vi "Error Query.vi"(8 "error in (no error)":errorcluster, 11 "VISA resource name":refnum<visa-resource-name>) -> (0 "error out":errorcluster, 1 "Error Message":string, 2 "Error Code":i32[](array[numeric]), 3 "VISA resource name out":refnum<visa-resource-name>)   [LabVIEW 2018, in "Tektronix TDS 200 1000 2000 Series.lvlib"]
doc: "Queries an instrument for any errors in the error queue of the instrument. The Error Query VI continuously reads errors until this VI reads all the errors from the instrument. \n<B>Note</B>: Because most driver VIs automatically call the Error Query VI, you do not need to call this VI in an application."
uses:
  Tektronix TDS 200 1000 2000 Series.lvlib
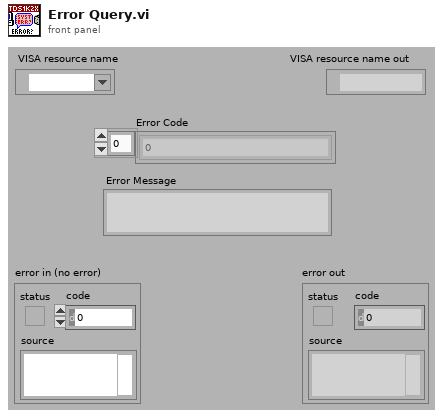
[diagram p1: front panel]
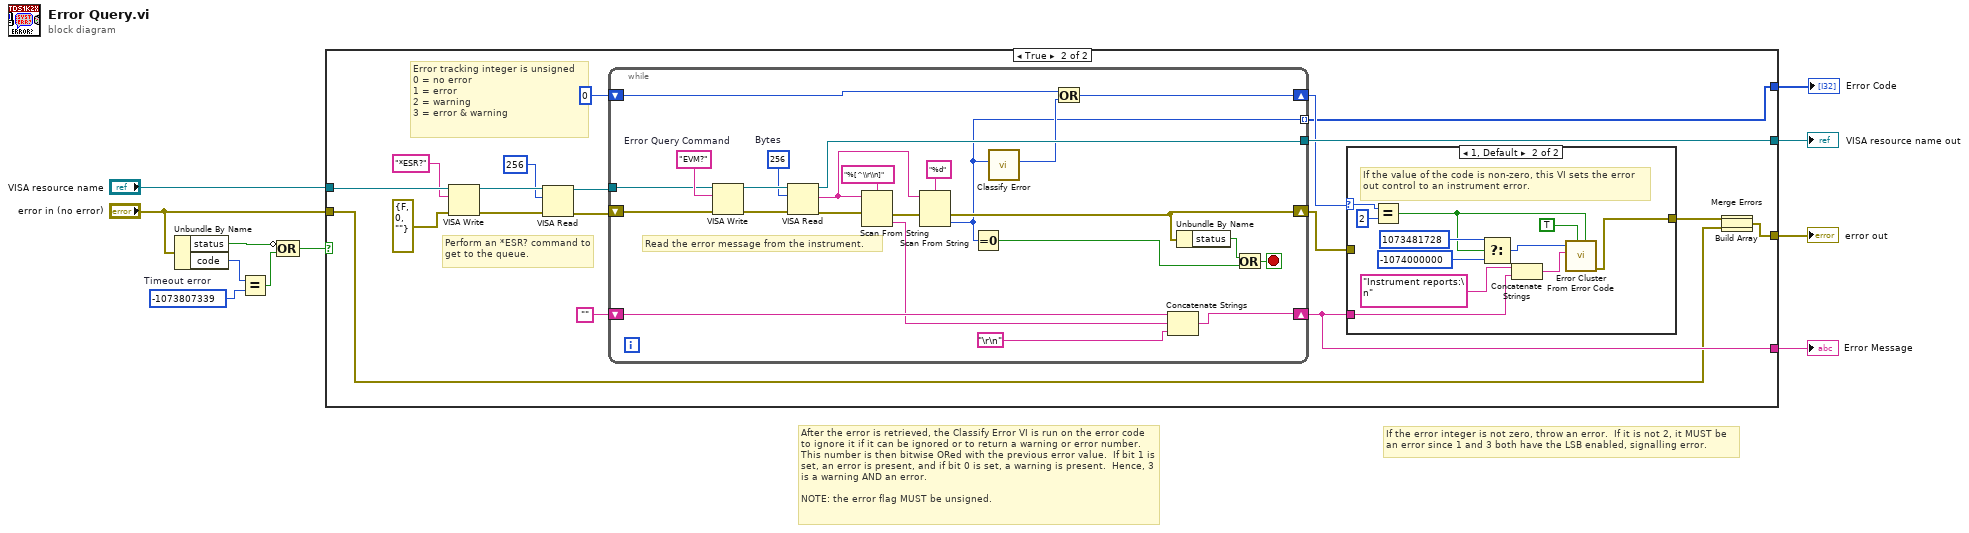
[diagram p0: block diagram]
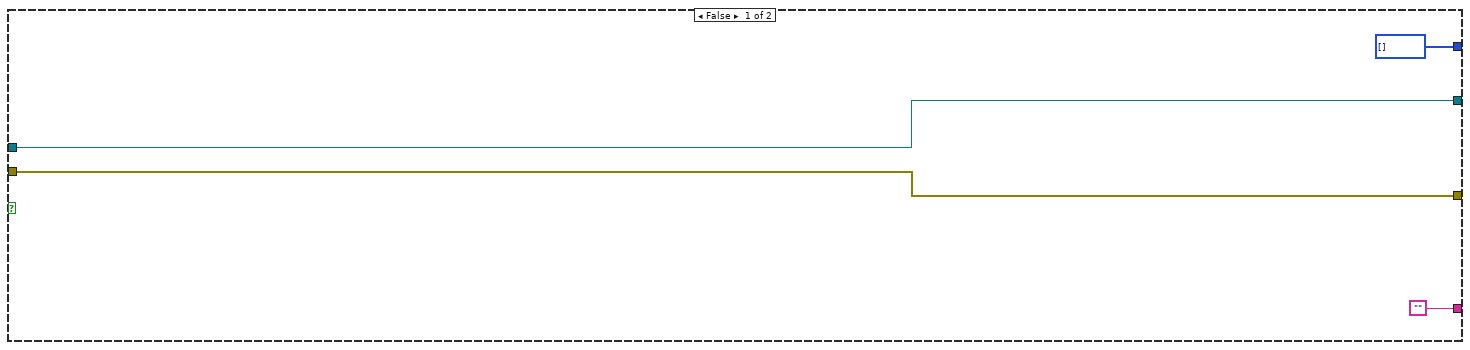
[diagram p2: hidden frame]
diagram:
  w6 = -1073807339  # Timeout error
  # "If the error integer is not zero, throw an error.  If it is not 2, it MUST be an error since 1 and 3 both have the LSB enabled, signalling error."
  # "After the error is retrieved, the Classify Error VI is run on the error code to ignore it if it can be ignored or to return a warning or error number.  This number is then bitwise ORed with the previous error value.  If bit 1 is set, an error is present, and if bit 0 is set, a warning is present.  Hence, 3 is a warning AND an error.\n\nNOTE: the error flag MUST be unsigned."
  n1 = Unbundle By Name("error in (no error)") -> ("status"=w7:bool, "code"=w4:i32)
  n2 = Equal?(x=w4, y=w6) -> (x = y?=w5:bool)
  n3 = Compound Arithmetic op=OR(invert w7, w5) -> (w3:bool)
  n4 = case shown="True" w3 {
    tunnel: [w15 w34] -> w11
    tunnel: "VISA resource name" -> [w15 w29]
    tunnel: "error in (no error)" -> [w14 w23]
    tunnel: [w14 w32] -> w9
    tunnel: ["" w30] -> w2
    tunnel: [i32[] [] w17] -> w1
    frame False {
    }
    frame True {
      # "Error tracking integer is unsigned\n0 = no error\n1 = error\n2 = warning\n3 = error & warning"
      # "Perform an *ESR? command to get to the queue."
      n5 = VISA Write(VISA resource name=w29, write buffer="*ESR?", error in (no error)=errorcluster {"status"=FALSE, "code"=0, "source"=""}) -> (VISA resource name out=w26:refnum<visa-resource-name>, error out=w27:errorcluster)  [unwired: 1 out]
      n6 = VISA Read(VISA resource name=w26, byte count=u32 256, error in (no error)=w27) -> (VISA resource name out=w24:refnum<visa-resource-name>, error out=w22:errorcluster)  [unwired: 2 out]
      n7 = while {
        tunnel: [w70] -> w34
        tunnel: w24 -> [w53]
        shift-right: [w59] -> w30
        shift-left: "" -> [w61]
        shift-right: [w50] -> w20
        shift-left: u32 0 ("x = 0?") -> [w49]
        shift-right: [w57] -> w19
        shift-left: w22 -> [w58]
        tunnel: [w47] -> w17 mode=indexing
        stop <- w64 stop-if-true
        w68 = u32 256  # Bytes
        w66 = "EVM?"  # Error Query Command
        # "Read the error message from the instrument."
        n8 = VISA Write(VISA resource name=w53, write buffer=w66, error in (no error)=w58) -> (VISA resource name out=w69:refnum<visa-resource-name>, error out=w67:errorcluster)  [unwired: 1 out]
        n9 = VISA Read(VISA resource name=w69, byte count=w68, error in (no error)=w67) -> (VISA resource name out=w70:refnum<visa-resource-name>, read buffer=w62:string, error out=w56:errorcluster)  [unwired: 1 out]
        n10 = Scan From String(format string="%[^\\r\\n]", input string=w62, error in=w56) -> (error out=w55:errorcluster, output 1=w60:string)  [unwired: 1 in, 3 out]
        n11 = Scan From String(format string="%d", input string=w62, error in=w55) -> (error out=w57:errorcluster, output 1=w47:i32)  [unwired: 1 in, 3 out]
        n12 = Equal To 0?(x=w47) -> (x = 0?=w52:bool)
        n13 = call "Classify Error.vi"("Error Code"=w47) -> ("Error Classification"=w48:u32)  [unwired: 10 out]
        n14 = Or(x=w49, y=w48) -> (x .or. y?=w50:u32)
        n15 = Concatenate Strings(w61, w60, "\r\n") -> (w59:string)
        n16 = Unbundle By Name(w57) -> ("status"=w54:bool)
        n17 = Or(x=w54, y=w52) -> (x .or. y?=w64:bool)
      }
      n18 = case shown="1, Default" w20 {
        selector: w20 -> [_ w41]
        tunnel: [w35 w42] -> w31
        tunnel: w30 -> [_ w43]
        tunnel: w19 -> [w35 _]
        frame 0 {
        }
        frame 1, Default {
          # "If the value of the code is non-zero, this VI sets the error out control to an instrument error."
          n19 = Equal?(x=w41, y=u32 2) -> (x = y?=w38:bool)
          n20 = Select(t=1073481728 ("Code"), s=w38, f=-1074000000 ("Code")) -> (s? t:f=w36:i32)
          n21 = Concatenate Strings("Instrument reports:\n" ("Source"), w43) -> (w44:string)
          n22 = call "Error Cluster From Error Code.vi"("is warning? (False)"=w38, "show call chain? (False)"=TRUE, "error message (\"\")"=w44, "error code (0)"=w36) -> ("error out"=w42:errorcluster)  [unwired: 1 in, 4 out]
        }
      }
      n23 = Build Array(w31, w23) -> (w16:errorcluster[])
      n24 = Merge Errors(w16) -> (w32:errorcluster)
    }
  }
  "VISA resource name out" <- w11
  "error out" <- w9
  "Error Message" <- w2
  "Error Code" <- w1
